vi "Scripting compiler.vi"() -> ()   [LabVIEW 2013]
uses:
  Command Type.ctl
  Robot Global Data.vi
panel:
  in  "error in":errorcluster
  out "error out":errorcluster
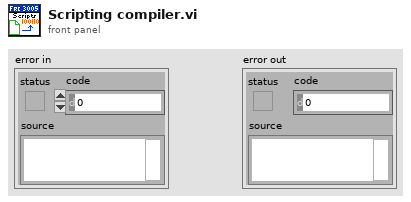
[diagram p1: front panel]
types:
  T1 = typedef "Command Type.ctl" = cluster{"Function Name":string, "Arguments":string[]}
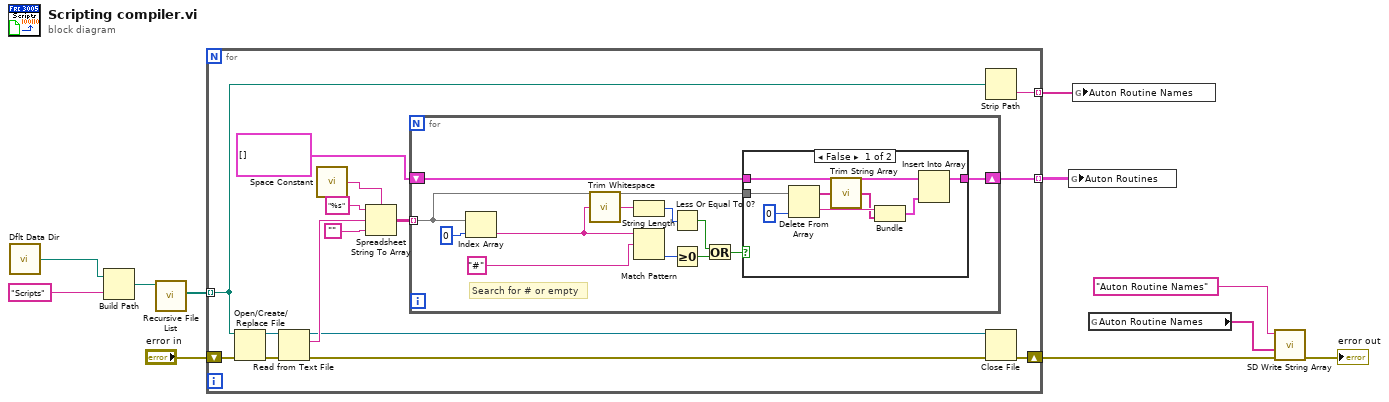
[diagram p0: block diagram]
diagram:
  n1 = call <vilib>:"Dflt Data Dir.vi"() -> ("App:Default Data Directory"=w9:path)
  n2 = Build Path(base path=w9, name or relative path="Scripts") -> (appended path=w10:path)
  n3 = call <vilib>:"Recursive File List.vi"("Folder Path"=w10) -> ("All Files in Dir"=w7:path[])  [unwired: 6 in, 4 out]
  n4 = for {
    shift-right: [w20] -> w2
    shift-left: "error in" -> [w19]
    tunnel: [w14] -> w6 mode=indexing
    tunnel: w7 -> [w13] mode=indexing
    tunnel: [w12] -> w8 mode=indexing
    n5 = Open/Create/Replace File(file path (use dialog)=w13, error in=w19) -> (refnum out=w25:refnum<file>, error out=w26:errorcluster)  [unwired: 4 in, 1 out]
    n6 = Read from Text File(file (use dialog)=w25, error in=w26) -> (refnum out=w17:refnum<file>, text=w24:string, error out=w21:errorcluster)  [unwired: 2 in, 1 out]
    n7 = call <vilib>:"Space Constant.vi"() -> ("String"=w22:string)
    n8 = Spreadsheet String To Array(delimiter (Tab)=w22, format string="%s", spreadsheet string=w24, array type (2D Dbl)="") -> (array=w18:string[][])
    n9 = for {
      tunnel: w18 -> [w28] mode=indexing
      shift-right: [w29] -> w14
      shift-left: T1[] [] ("Auton Routine") -> [w36]
      # "Search for # or empty"
      n10 = Index Array(array=w28, index=0) -> (element=w33:string)
      n11 = call <vilib>:"Trim Whitespace.vi"("string"=w33) -> ("trimmed string"=w27:string)  [unwired: 1 in]
      n12 = String Length(string=w27) -> (length=w34:i32)
      n13 = Match Pattern(string=w33, regular expression="#") -> (offset past match=w35:i32)  [unwired: 1 in, 3 out]
      n14 = Less Or Equal To 0?(x=w34) -> (x <= 0?=w30:bool)
      n15 = Greater Or Equal To 0?(x=w35) -> (x >= 0?=w31:bool)
      n16 = Or(x=w30, y=w31) -> (x .or. y?=w32:bool)
      n17 = case shown="False" w32 {
        tunnel: w36 -> [w43 w47]
        tunnel: [w42 w47] -> w29
        tunnel: w28 -> [w46 _]
        frame False {
          n18 = Delete From Array(array=w46, index=0) -> (deleted portion=w44:string, array with subset deleted=w41:string[])  [unwired: 1 in]
          n19 = call "Trim String Array.vi"("String Array"=w41) -> ("String Array Trimmed"=w40:string[])  [unwired: 14 in]
          n20 = Bundle(w44, "String Array Trimmed"=w40) -> (w39:cluster{string, "String Array Trimmed":string[]})  [unwired: 1 in]
          n21 = Insert Into Array(array=w43, new element=w39) -> (w42:T1[])  [unwired: 1 in]
        }
        frame True {
        }
      }
    }
    n22 = Strip Path(path=w13) -> (name=w12:string)  [unwired: 1 out]
    n23 = Close File(refnum=w17, error in=w21) -> (error out=w20:errorcluster)  [unwired: 1 out]
  }
  n24 = global write "Robot Global Data.vi" "Auton Routines"(w6) -> ()
  n25 = global write "Robot Global Data.vi" "Auton Routine Names"(w8) -> ()
  n26 = global read "Robot Global Data.vi" "Auton Routine Names"() -> (w3:string[])
  n27 = call <vilib>:"SD Write String Array.vi"("error in"=w2, "String Array"=w3, "Name"="Auton Routine Names") -> ("error out"=→"error out":errorcluster)  [unwired: 7 in, 1 out]
